vi "Index Array Elements (1D) Example 01.vi"() -> ()   [LabVIEW 2011]
uses:
  <userlib>/_OpenG.lib/array/array.llb/Index 1D Array Elements (String)__ogtk.vi
panel:
  out "elements":string[](array[string])
  in  "indices":i32[](array[numeric])=[0, 2]
  in  "array":string[](array[string])=["Blue", "Red", "Monkey", "Fish"]
  # "<== These are the indices of elements from array, that you want to obtain in the elements array."
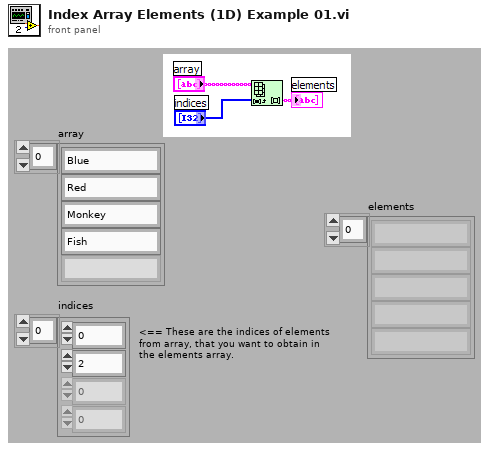
[diagram p1: front panel]
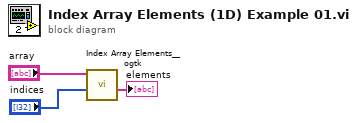
[diagram p0: block diagram]
diagram:
  n1 = call-poly <userlib>:"Index Array Elements__ogtk.vi"("indices"="indices", "array"="array") -> ("elements"=→"elements":string[])  [unwired: 9 in]
